vi "Validate Decimal Number.vi"(0 "String":string, 2 "Empty Default":dbl) -> (4 "Valid":bool, 5 "Value":dbl)   [LabVIEW 2020, in "VolatusGUIElements.lvlib" / "BluelinesRedlines.lvclass"]
uses:
  BluelinesRedlines.lvclass
  BluelinesRedlines.lvclass/BluelinesRedlines.ctl
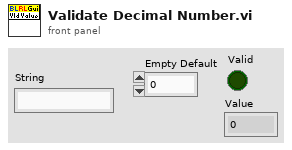
[diagram p1: front panel]
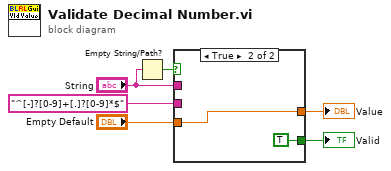
[diagram p0: block diagram]
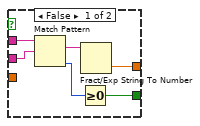
[diagram p2: hidden frame]
diagram:
  n1 = Empty String/Path?(string/path="String") -> (empty?=w1:bool)
  n2 = case shown="True" w1 {
    tunnel: "String" -> [w12 _]
    tunnel: "^[-]?[0-9]+[.]?[0-9]*$" -> [w11 _]
    tunnel: [w9 TRUE] -> w5
    tunnel: [w7 w14] -> w4
    tunnel: "Empty Default" -> [_ w14]
    frame False {
      n3 = Match Pattern(string=w12, regular expression=w11) -> (match substring=w8:string, offset past match=w10:i32)  [unwired: 1 in, 2 out]
      n4 = Greater Or Equal To 0?(x=w10) -> (x >= 0?=w9:bool)
      n5 = Fract/Exp String To Number(string=w8) -> (number=w7:dbl)  [unwired: 3 in, 1 out]
    }
    frame True {
    }
  }
  "Valid" <- w5
  "Value" <- w4
